vi "Xbox Layout.vi"(3 "Joystick Name":string) -> (0 "Center Left":bool, 7 "Arrows":i16, 8 "Center Right":bool, 9 "A":bool, 12 "Left Button":bool, 13 "B":bool, 14 "Right Button":bool, 15 "X":bool, 17 "Y":bool, 20 "Left Stick Y":dbl, 21 "Left Stick X":dbl, 22 "Left Throttle":bool, 23 "Left Stick Touch":bool, 24 "Right Stick Y":dbl, 25 "Right Stick X":dbl, 26 "Right Throttle":bool, 27 "Right Stick Touch":bool)   [LabVIEW 2015]
doc: "Outputs the values (Axes and Buttons) from an XBox controller."
uses:
  <vilib>/Rock Robotics/WPI/Utilities/WPI_GetSetVariantRefNum.vi
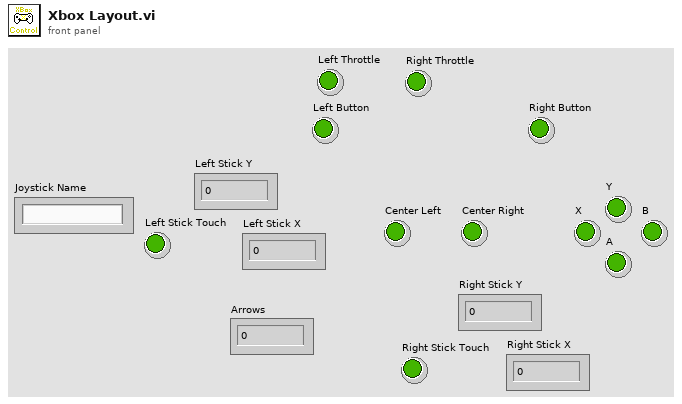
[diagram p1: front panel]
types:
  T1 = typedef "WPI_JoystickDevRef.ctl" = cluster{"Device":T2}
  T2 = typedef "WPI_JoystickDeviceEnum.ctl" = enum16{"USB 0", "USB 1", "USB 2", "USB 3", "USB 4", "USB 5"}
  T3 = cluster{"Button 1":bool, "Button 2":bool, "Button 3":bool, "Button 4":bool, "Button 5":bool, "Button 6":bool, "Button 7":bool, "Button 8":bool, "Button 9":bool, "Button 10":bool, "Button 11":bool, "Button 12":bool}
  T4 = cluster{"Axes[0]":dbl, "Axes[1]":dbl, "Axes[2]":dbl, "Axes[3]":dbl, "Axes[4]":dbl, "Axes[5]":dbl, "Axes[6]":dbl, "Axes[7]":dbl, "Axes[8]":dbl}
  T5 = cluster{"POVs[0]":i16, "POVs[1]":i16, "POVs[2]":i16, "POVs[3]":i16, "POVs[4]":i16, "POVs[5]":i16, "POVs[6]":i16, "POVs[7]":i16, "POVs[8]":i16}
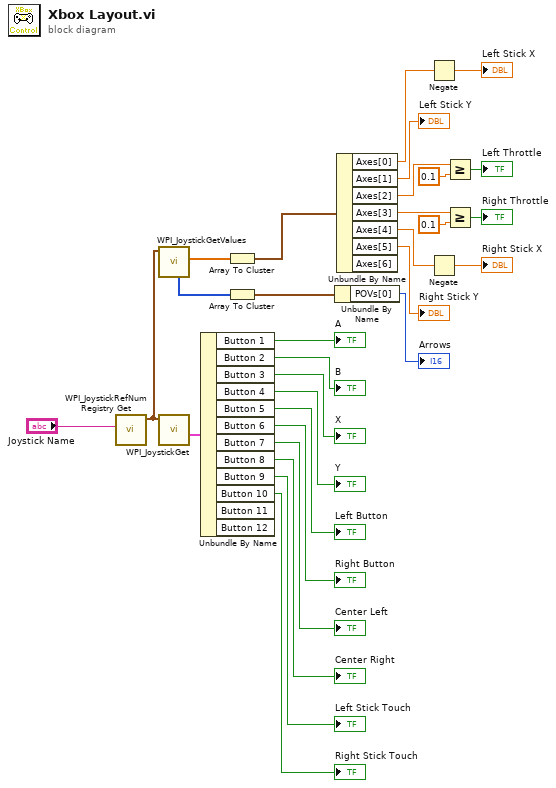
[diagram p0: block diagram]
diagram:
  n1 = call <vilib>:"WPI_JoystickRefNum Registry Get.vi"("refnum name"="Joystick Name") -> ("JoystickDevRef"=w14:T1)  [unwired: 9 in, 1 out]
  n2 = call <vilib>:"WPI_JoystickGetValues.vi"("JoystickDevRef"=w14) -> ("Axes"=w13:dbl[], "POVs"=w9:i16[])  [unwired: 6 in, 3 out]
  n3 = call <vilib>:"WPI_JoystickGet.vi"("JoystickDevRef"=w14) -> ("Buttons"=w29:T3)  [unwired: 4 in, 2 out]
  n4 = Unbundle By Name(w29) -> ("Button 1"=→"A":bool, "Button 2"=→"B":bool, "Button 3"=→"X":bool, "Button 4"=→"Y":bool, "Button 5"=→"Left Button":bool, "Button 6"=→"Right Button":bool, "Button 7"=→"Center Left":bool, "Button 8"=→"Center Right":bool, "Button 9"=→"Left Stick Touch":bool, "Button 10"=→"Right Stick Touch":bool)  [unwired: 2 out]
  n5 = Array To Cluster(array=w13) -> (cluster=w12:T4)
  n6 = Array To Cluster(array=w9) -> (cluster=w8:T5)
  n7 = Unbundle By Name(w8) -> ("POVs[0]"=→"Arrows":i16)
  n8 = Unbundle By Name(w12) -> ("Axes[0]"=w27:dbl, "Axes[1]"=→"Left Stick Y":dbl, "Axes[2]"=w6:dbl, "Axes[3]"=w1:dbl, "Axes[4]"=w11:dbl, "Axes[5]"=→"Right Stick Y":dbl)  [unwired: 1 out]
  n9 = Negate(x=w27) -> (-x=→"Left Stick X":dbl)
  n10 = Negate(x=w11) -> (-x=→"Right Stick X":dbl)
  n11 = Greater Or Equal?(x=w6, y=0.1) -> (x >= y?=→"Left Throttle":bool)
  n12 = Greater Or Equal?(x=w1, y=0.1) -> (x >= y?=→"Right Throttle":bool)
